vi "dfd_Direct_IIR_II_T_C.vi"() -> ()   [LabVIEW 2017, in "NI_DigFilterTemp.lvlib"]
uses:
  <vilib>/addons/Digital Filter Design/NI_DigFilterTemp.lvlib
panel:
  in  "String":string="\n\n/* ---- Constants ----*/\n#define %CapName%_N_STATES %kIIRStatesAmt%\n#define %CapName%_N_COEFA %kCoefsAAmt%\n#define %CapName%_N_COEFB %kCoefsBAmt%\n\n/* ---- Global Variables Declaration ----*/\nstatic %CoefAType% %FilterBlkName%_CoefA[%CapName%_N_COEFA];\nstatic %CoefBType% %FilterBlkName%_CoefB[%CapName%_N_COEFB];\n%InternalFunctionsDeclaration%\n\n%ShiftDefine%\n\n%AssistantFunctions%\n\n/* ---- Implement the Fixed-Point Filter ---- */\n%OutType% %FilterBlkName%_Filtering (%InType% sampleIn, %FilterBlkName%_State state)\n{\n\tI32 accA, accB;\n\t%InType% mult_b;\n\t%MultType% mult_a;\n\tint i;\n\t\n\tmult_b = sampleIn;\n\n\t/* Filtering */\n\taccA = (%FilterBlkName%_%MultB%(mult_b, %FilterBlkName%_CoefB[0]) << PROD2SUM);\n\taccA += (state[0] << DELAY2SUM);\n\n\t/* Update the internal states */\n\tfor (i=0; i < (%CapName%_N_STATES-1); i++)\n\t\tstate[i] = state[i+1];\n\tstate[i] = 0;\n\n\tfor (i=1; i < %CapName%_N_COEFB; i++)\n\t{\n\t\taccB = (%FilterBlkName%_%MultB%(mult_b, %FilterBlkName%_CoefB[i]) << PROD2SUM);\n\t\taccB += (state[i-1] << DELAY2SUM);\n\t\tstate[i-1] = (accB << SUM2DELAY);\n\t}\n\n\tmult_a = %PreMultCast%(accA << SUM2MULT);\n\n\tfor (i=0; i < %CapName%_N_COEFA; i++)\n\t{\n\t\taccB = (%FilterBlkName%_%MultA%(mult_a, %FilterBlkName%_CoefA[i]) << PROD2SUM);\n\t\taccB = (state[i] << DELAY2SUM) - accB;\n\t\tstate[i] = (accB << SUM2DELAY);\n\t}\n\n\t%ApplyGainAccA%\n\n\treturn (%OutType%)accA;\n}\n\n/* ---- Internal Functions ---- */\n%InternalFunctions%\n\n/* ---- Filter Coefficients ---- */\nstatic %CoefAType% %FilterBlkName%_CoefA [] = {\n%CoefficientsA%\n};\nstatic %CoefBType% %FilterBlkName%_CoefB [] = {\n%CoefficientsB%\n};\n"
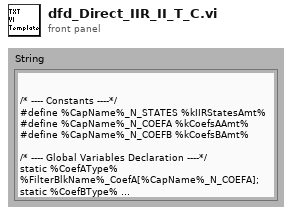
[diagram p1: front panel]
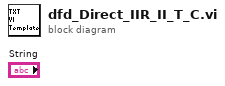
[diagram p0: block diagram]
diagram:
